vi "Get Specific Filter Configuration String.vi"(11 "String Filters in":refnum<class "String Filters.lvclass">) -> (2 "Filter String":string)   [LabVIEW 2016, in "Assert API Components.lvlib" / "String Filters.lvclass"]
uses:
  String Filters.lvclass
  String Filters.lvclass/String Filters.ctl
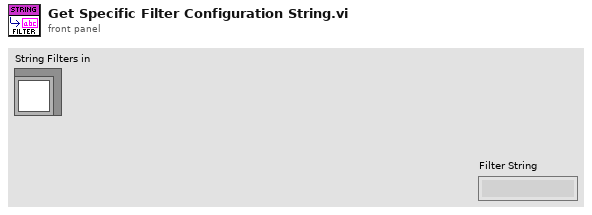
[diagram p1: front panel]
types:
  T1 = enum16{"Contains", "Does Not Contain", "Starts With", "Equals", "Does Not Equal"}
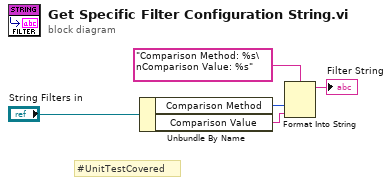
[diagram p0: block diagram]
diagram:
  # "#UnitTestCovered"
  n1 = Unbundle By Name("String Filters in") -> ("Comparison Method"=w3:T1, "Comparison Value"=w2:string)
  n2 = Format Into String(format string="Comparison Method: %s\nComparison Value: %s", w3, w2) -> (resulting string=→"Filter String":string)  [unwired: 2 in, 1 out]
